vi "营养盐XML解析.vi"(10 "启动模式":enum16{"水样测量", "零液测量", "标液测量"}(ring), 11 "启动参数":T1(ring)) -> (2 "步骤时间":string[](array[string]), 3 "步骤名":string[](array[string]))   [LabVIEW 2016]
uses:
  <vilib>/Utility/sysdir.llb/System Directory Type.ctl
  <vilib>/xml/Load XML File.vi
  <vilib>/xml/Close Reference(Node).vi
  <resource>/objmgr/DOMUserDefRef.rc
  <vilib>/xml/NI_XML.lvlib
panel:
  out "添加的路径":path
  out "XML字符串":string="<?xml version=\"1.0\" encoding=\"ISO-8859-1\"?>\n<bookstore>\n<book ISBN=\"978-0545128285\">\n  <title lang=\"en\">The Tales of Beedle the Bard</title>\n  <author>J. K. Rowling</author>\n  <year>2008</year>\n  <price>12.99</price>\n</book>\n<book ISBN=\"978-0316160209\">\n  <title lang=\"en\">Eclipse</title>\n  <author>Stephenie Meyer</author>\n  <year>2007</year>\n  <price>19.99</price>\n</book>\n<book ISBN=\"978-0316067928\">\n  <title lang=\"en\">Breaking Dawn</title>\n  <author>Stephenie Meyer</author>\n  <year>2008</year>\n  <price>22.99</price>\n</book>\n<book ISBN=\"978-0316017923\">\n  <title lang=\"en\">Outliers: The Story of Success</title>\n  <author>Malcolm Gladwell</author>\n  <year>2008</year>\n  <price>27.99</price>\n</book>\n<book ISBN=\"978-0596007645\">\n  <title lang=\"en\">XML in a Nutshell</title>\n  <author>Elliotte Rusty Harold</author>\n  <author>W. Scott Means</author>\n  <year>2004</year>\n  <price>39.95</price>\n</book>\n</bookstore>"
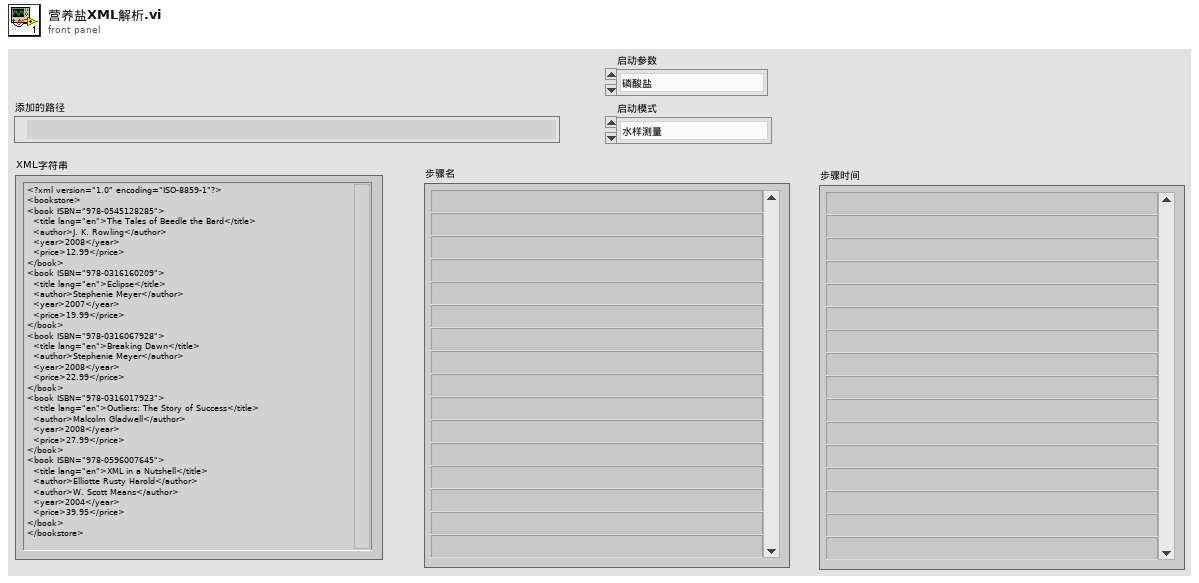
[diagram p1: front panel]
types:
  T1 = enum16{"磷酸盐", "亚硝酸盐", "硫化物", "硝氮", "OPA", "填充试剂"}
  T2 = typedef "System Directory Type.ctl" = i32
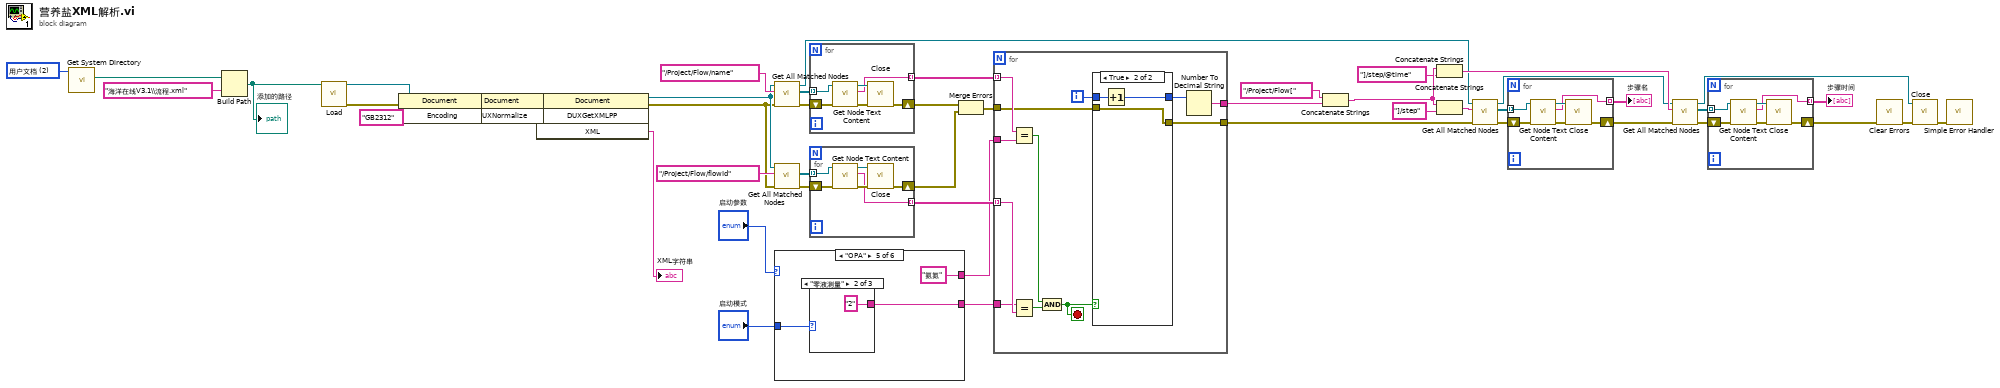
[diagram p0: block diagram]
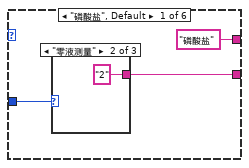
[diagram p2: hidden frame]
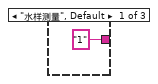
[diagram p3: hidden frame]
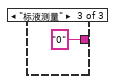
[diagram p4: hidden frame]
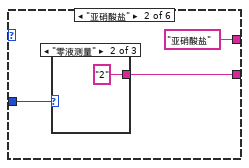
[diagram p5: hidden frame]
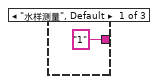
[diagram p6: hidden frame]
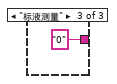
[diagram p7: hidden frame]
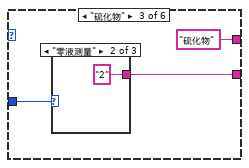
[diagram p8: hidden frame]
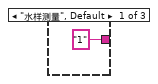
[diagram p9: hidden frame]
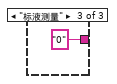
[diagram p10: hidden frame]
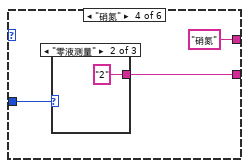
[diagram p11: hidden frame]
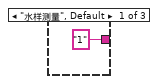
[diagram p12: hidden frame]
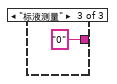
[diagram p13: hidden frame]
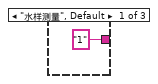
[diagram p14: hidden frame]
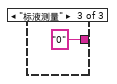
[diagram p15: hidden frame]
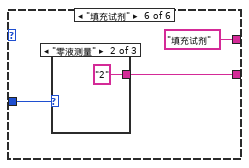
[diagram p16: hidden frame]
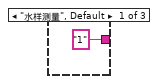
[diagram p17: hidden frame]
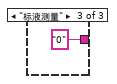
[diagram p18: hidden frame]
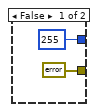
[diagram p19: hidden frame]
diagram:
  w27 = T2 2 items=["用户目录"=0, "用户桌面"=1, "用户文档"=2, "用户应用程序数据"=3, "用户设置"=4, "用户临时目录"=5, "公共文档"=6, "公共应用程序数据"=7, "公共设置"=8, "公共缓存"=13, "系统核心库"=9, "系统安装库"=10, "应用程序文件"=11, "启动盘根目录"=12] ("system directory type")
  n1 = call <vilib>:"Get System Directory.vi"("system directory type"=w27) -> ("system directory"=w26:path)  [unwired: 10 in]
  n2 = Build Path(base path=w26, name or relative path="海洋在线V3.1\\流程.xml" ("名称或相对路径")) -> (appended path=w24:path)
  "添加的路径" <- w24
  n3 = call-poly <vilib>:"Load.vi"("path to XML document"=w24) -> ("DOM document out"=w47:refnum<k20>, "error out"=w46:errorcluster)  [unwired: 12 in, 1 out]
  n4 = property on="属性节点" class="Document"(reference=w47, error in=w46, "Encoding"="GB2312" ("文档编码")) -> (reference out=w44:refnum<k20>, error out=w43:errorcluster)
  n5 = invoke on="Invoke Node" class="Document" method="DUXNormalize"(reference=w44, error in=w43) -> (reference out=w41:refnum<k20>, error out=w42:errorcluster)  [unwired: 1 in, 1 out]
  n6 = invoke on="Invoke Node" class="Document" method="DUXGetXMLPP"(reference=w41, error in=w42) -> (reference out=w17:refnum<k20>, error out=w16:errorcluster, "XML"=→"XML字符串":string)  [unwired: 2 in, 1 out]
  n7 = call <vilib>:"Get All Matched Nodes.vi"("error in (no error)"=w16, "XPath expression"="/Project/Flow/name", "node in"=w17) -> ("error out"=w13:errorcluster, "node result array"=w22:refnum<k20>[], "node out"=w14:refnum<k20>)  [unwired: 6 out]
  n8 = call <vilib>:"Get All Matched Nodes.vi"("error in (no error)"=w16, "XPath expression"="/Project/Flow/flowId", "node in"=w17) -> ("error out"=w12:errorcluster, "node result array"=w20:refnum<k20>[])  [unwired: 7 out]
  n9 = case shown="\"OPA\"" "启动参数" {
    tunnel: "启动模式" -> [w53 w58 w64 w71 w77 w82]
    tunnel: [w52 w57 w65 w69 w75 w81] -> w2
    tunnel: ["磷酸盐" "亚硝酸盐" "硫化物" "硝氮" "氨氮" "填充试剂"] -> w1
    frame "磷酸盐", Default {
      n10 = case shown="\"零液测量\"" w53 {
        tunnel: ["1" "2" "0"] -> w52
        frame "水样测量", Default {
        }
        frame "零液测量" {
        }
        frame "标液测量" {
        }
      }
    }
    frame "亚硝酸盐" {
      n11 = case shown="\"零液测量\"" w58 {
        tunnel: ["1" "2" "0"] -> w57
        frame "水样测量", Default {
        }
        frame "零液测量" {
        }
        frame "标液测量" {
        }
      }
    }
    frame "硫化物" {
      n12 = case shown="\"零液测量\"" w64 {
        tunnel: ["1" "2" "0"] -> w65
        frame "水样测量", Default {
        }
        frame "零液测量" {
        }
        frame "标液测量" {
        }
      }
    }
    frame "硝氮" {
      n13 = case shown="\"零液测量\"" w71 {
        tunnel: ["1" "2" "0"] -> w69
        frame "水样测量", Default {
        }
        frame "零液测量" {
        }
        frame "标液测量" {
        }
      }
    }
    frame "OPA" {
      n14 = case shown="\"零液测量\"" w77 {
        tunnel: ["1" "2" "0"] -> w75
        frame "水样测量", Default {
        }
        frame "零液测量" {
        }
        frame "标液测量" {
        }
      }
    }
    frame "填充试剂" {
      n15 = case shown="\"零液测量\"" w82 {
        tunnel: ["1" "2" "0"] -> w81
        frame "水样测量", Default {
        }
        frame "零液测量" {
        }
        frame "标液测量" {
        }
      }
    }
  }
  n16 = for {
    tunnel: w22 -> [w91] mode=indexing
    shift-right: [w92] -> w10
    shift-left: w13 -> [w90]
    tunnel: [w87] -> w21 mode=indexing
    n17 = call <vilib>:"Get Node Text Content.vi"("error in (no error)"=w90, "node in"=w91) -> ("error out"=w88:errorcluster, "node text"=w87:string, "node out"=w89:refnum<k20>)  [unwired: 7 in]
    n18 = call-poly <vilib>:"Close.vi"("error in (no error)"=w88, "node"=w89) -> ("error out"=w92:errorcluster)  [unwired: 7 out]
  }
  n19 = for {
    shift-right: [w98] -> w11
    shift-left: w12 -> [w97]
    tunnel: [w94] -> w18 mode=indexing
    tunnel: w20 -> [w93] mode=indexing
    n20 = call <vilib>:"Get Node Text Content.vi"("error in (no error)"=w97, "node in"=w93) -> ("error out"=w95:errorcluster, "node text"=w94:string, "node out"=w96:refnum<k20>)  [unwired: 7 in]
    n21 = call-poly <vilib>:"Close.vi"("error in (no error)"=w95, "node"=w96) -> ("error out"=w98:errorcluster)  [unwired: 7 out]
  }
  n22 = Merge Errors(w10, w11) -> (w9:errorcluster)
  n23 = for {
    tunnel: w21 -> [w110] mode=indexing
    tunnel: w18 -> [w109] mode=indexing
    tunnel: [w103] -> w15
    tunnel: w1 -> [w102]
    tunnel: w2 -> [w101]
    tunnel: w9 -> [w100]
    tunnel: [w99] -> w8
    i -> [w105]
    stop <- w106 stop-if-true
    n24 = Equal?(x=w110, y=w102) -> (x = y?=w107:bool)
    n25 = Equal?(x=w101, y=w109) -> (x = y?=w108:bool)
    n26 = And(x=w107, y=w108) -> (x .and. y?=w106:bool)
    n27 = case shown="True" w106 {
      tunnel: w105 -> [_ w114]
      tunnel: [255 w113] -> w104
      tunnel: w100 -> [_ w115]
      tunnel: [errorcluster {"status"=TRUE, "code"=0, "source"=""} ("错误常量") w115] -> w99
      frame False {
      }
      frame True {
        n28 = Increment(x=w114) -> (x+1=w113:i32)
      }
    }
    n29 = Number To Decimal String(number=w104) -> (decimal integer string=w103:string)  [unwired: 1 in]
  }
  n30 = Concatenate Strings("/Project/Flow[" ("XPath expression"), w15) -> (w34:string)
  n31 = Concatenate Strings(w34, "]/step/@time" ("XPath expression")) -> (w32:string)
  n32 = Concatenate Strings(w34, "]/step" ("XPath expression")) -> (w35:string)
  n33 = call <vilib>:"Get All Matched Nodes.vi"("error in (no error)"=w8, "XPath expression"=w35, "node in"=w14) -> ("error out"=w50:errorcluster, "node result array"=w45:refnum<k20>[], "node out"=w30:refnum<k20>)  [unwired: 6 out]
  n34 = for {
    tunnel: w45 -> [w120] mode=indexing
    shift-right: [w121] -> w38
    shift-left: w50 -> [w119]
    tunnel: [w116] -> w40 mode=indexing
    n35 = call <vilib>:"Get Node Text Content.vi"("error in (no error)"=w119, "node in"=w120) -> ("error out"=w117:errorcluster, "node text"=w116:string, "node out"=w118:refnum<k20>)  [unwired: 7 in]
    n36 = call-poly <vilib>:"Close.vi"("error in (no error)"=w117, "node"=w118) -> ("error out"=w121:errorcluster)  [unwired: 7 out]
  }
  "步骤名" <- w40
  n37 = call <vilib>:"Get All Matched Nodes.vi"("error in (no error)"=w38, "XPath expression"=w32, "node in"=w30) -> ("error out"=w37:errorcluster, "node result array"=w31:refnum<k20>[], "node out"=w29:refnum<k20>)  [unwired: 6 out]
  n38 = for {
    tunnel: w31 -> [w126] mode=indexing
    shift-right: [w127] -> w6
    shift-left: w37 -> [w125]
    tunnel: [w122] -> w28 mode=indexing
    n39 = call <vilib>:"Get Node Text Content.vi"("error in (no error)"=w125, "node in"=w126) -> ("error out"=w123:errorcluster, "node text"=w122:string, "node out"=w124:refnum<k20>)  [unwired: 7 in]
    n40 = call-poly <vilib>:"Close.vi"("error in (no error)"=w123, "node"=w124) -> ("error out"=w127:errorcluster)  [unwired: 7 out]
  }
  "步骤时间" <- w28
  n41 = call <vilib>:"Clear Errors.vi"("error in (no error)"=w6) -> ("error out"=w5:errorcluster)  [unwired: 5 in, 1 out]
  n42 = call-poly <vilib>:"Close.vi"("error in (no error)"=w5, "node"=w29) -> ("error out"=w7:errorcluster)  [unwired: 7 out]
  n43 = call <vilib>:"Simple Error Handler.vi"("error in (no error)"=w7) -> ()  [unwired: 4 in, 5 out]
